vi "Change AO Gain On Fly.vi"() -> ()   [LabVIEW 2015]
doc: "I. Description:\nThis example demonstrates how to output a continuous periodic waveform using an internal sample clock.\n\nII. Instructions for Running:\n1. Select the Physical Channel to correspond to where your signal is output on the DAQ device.\n2. Enter the Minimum and Maximum Voltage Ranges\n3. Specify the Desired Frequency of the output Waveform\n4. Enter the Waveform Information. See the documentation of the Waveform Buffer Generation SubVI for information on each parameter.\n\nIII. Block Diagram Steps:\n1. Create an Analog Output Voltage channel.\n2. Call the DAQmx Timing (Use Waveform) VI which sets the sample clock rate based on the input waveform parameters, and set the sample mode to Continuous.\n3. Write the waveform to the output buffer.\n4. Call the Start VI.\n5. Loop continuously until the user presses the Stop button. Check for errors every 100 ms using the Is Task Done? VI\n6. Clear the Task\n7. Use the popup dialog box to display an error or warning if any.\n\nIV. I/O Connections Overview:\nMake sure your signal output terminal matches the Physical Channel I/O Control. For further connection information, refer to your hardware reference manual."
uses:
  <vilib>/DAQmx/create/channels.llb/DAQmx Create Channel (AO-Voltage-Basic).vi
  <vilib>/Utility/error.llb/DialogType.ctl
  <vilib>/DAQmx/configure/timing.llb/DAQmx Timing (Sample Clock).vi
  <vilib>/DAQmx/write.llb/DAQmx Write (Analog 2D I32 NChan NSamp).vi
panel:
  in  "AO Channel":u16(ring)=1536 items=["AO 0"=1536, "AO 1"=1540]
  in  "Gain Setting":u16(ring) items=["0 dB Gain"=0, "20 dB Gain"=2, "40 dB Gain"=4]
  out "Resulting Frequency":dbl format="%.2f"
  in  "Cycles per Buffer":i32=5
  in  "Waveform Type":T1(ring)
  in  "Desired Frequency":dbl=1000.0 format="%.2f"
  in  "Samples per Buffer":dbl=250.0
  in  "Amplitude":dbl=1750000000.0 format="%0.2p"
  out "Waveform Graph":i32[](graph) caption="Output Waveform"
  in  "Physical Channels":tag="PXI1Slot2/ao0:1"
  in  "Minimum Value":dbl=-10.0 format="%0.2f"
  in  "Maximum Value":dbl=10.0 format="%0.2f"
  in  "stop":bool
  # "For instructions, select Help>>Show Context Help"
  # "Channel Parameters"
  # "Timing Parameters"
  # "Waveform Information"
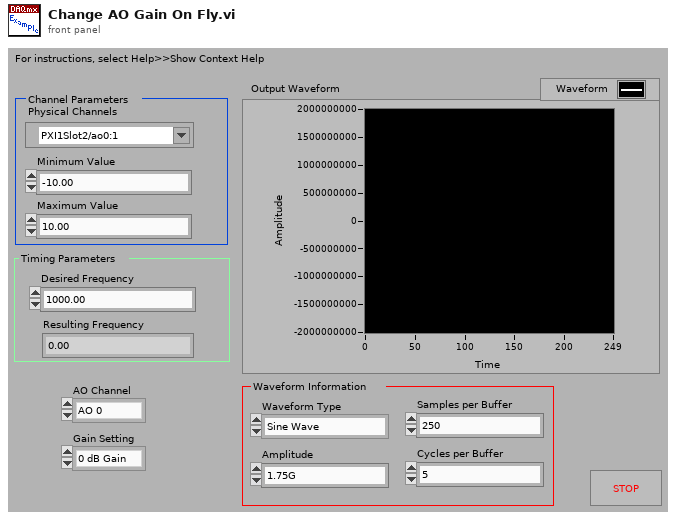
[diagram p1: front panel]
types:
  T1 = enum16{"Sine Wave", "Triangle Wave", "Square Wave", "Sawtooth Wave"}
  T2 = typedef "DialogType.ctl" = u16
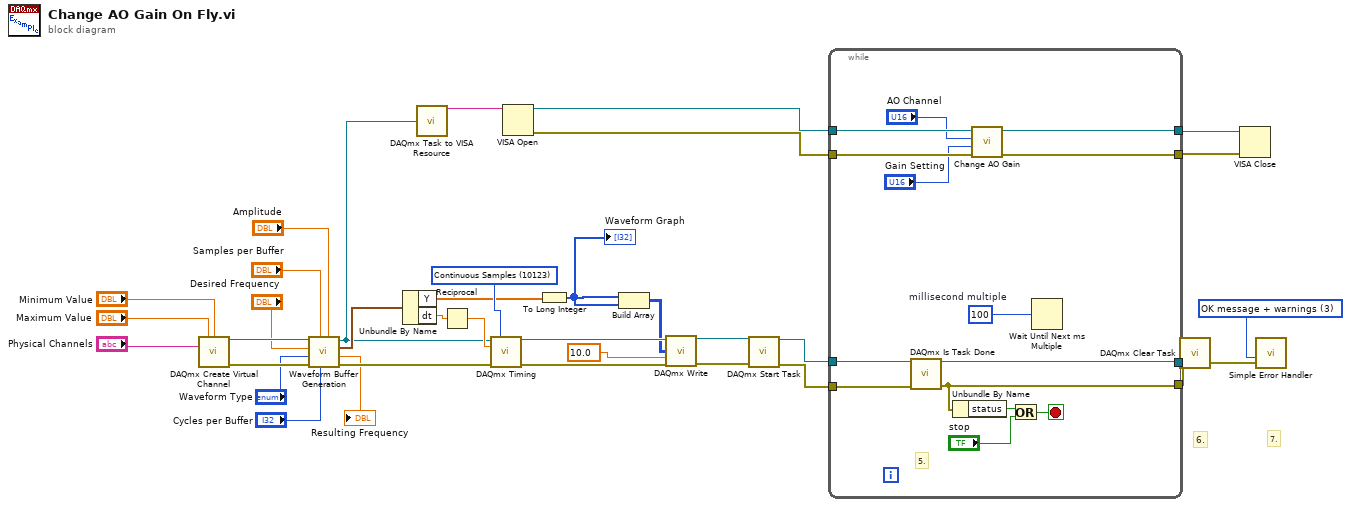
[diagram p0: block diagram]
diagram:
  w6 = 10123 items=["Finite Samples"=10178, "Continuous Samples"=10123, "Hardware Timed Single Point"=12522] ("sample mode")
  w25 = T2 3 items=["no dialog", "OK message", "continue or stop message", "OK message + warnings", "continue/stop + warnings"] ("type of dialog (OK msg:1)")
  # "7."
  # "6."
  n1 = call-poly <vilib>:"DAQmx Create Virtual Channel.vi"("maximum value"="Maximum Value", "minimum value"="Minimum Value", "physical channels"="Physical Channels") -> ("task out"=w21:refnum<k21>, "error out"=w20:errorcluster)  [unwired: 11 in]
  n2 = call "Waveform Buffer Generation.vi"("Amplitude"="Amplitude", "Cycles per Buffer"="Cycles per Buffer", "Samples per Buffer"="Samples per Buffer", "error in (no error)"=w20, "Waveform Type"="Waveform Type", "Desired Frequency"="Desired Frequency", "task/channels in"=w21) -> ("error out"=w22:errorcluster, "Resulting Frequency"=→"Resulting Frequency":dbl, "Waveform"=w9:waveform(dbl), "task out"=w1:refnum<k21>)  [unwired: 1 out]
  n3 = Unbundle By Name(w9) -> ("Y"=w2:dbl[], "dt"=w8:dbl)
  n4 = call "DAQmx Task to VISA Resource.vi"("task out"=w1) -> ("VISAName"=w14:string)
  n5 = Reciprocal(x=w8) -> (1/x=w7:dbl)
  n6 = call-poly <vilib>:"DAQmx Timing.vi"("task/channels in"=w1, "sample mode"=w6, "rate"=w7, "error in"=w22) -> ("task out"=w28:refnum<k21>, "error out"=w27:errorcluster)  [unwired: 10 in]
  n7 = VISA Open(VISA resource name=w14) -> (VISA resource name=w13:refnum<visa-resource-name>, error out=w12:errorcluster)  [unwired: 4 in]
  n8 = To Long Integer(number=w2) -> (32bit integer=w3:i32[])
  "Waveform Graph" <- w3
  n9 = Build Array(w3, w3) -> (w5:i32[][])
  n10 = call-poly <vilib>:"DAQmx Write.vi"("task/channels in"=w28, "data"=w5, "timeout"=10.0 ("Wirite Timeout"), "error in"=w27) -> ("task out"=w33:refnum<k21>, "error out"=w32:errorcluster)  [unwired: 9 in, 1 out]
  n11 = call <vilib>:"DAQmx Start Task.vi"("task/channels in"=w33, "error in"=w32) -> ("task out"=w26:refnum<k21>, "error out"=w30:errorcluster)  [unwired: 12 in]
  n12 = while {
    tunnel: w26 -> [w50]
    tunnel: [w49] -> w24
    tunnel: w30 -> [w48]
    tunnel: [w47] -> w23
    tunnel: w13 -> [w42]
    tunnel: w12 -> [w41]
    tunnel: [w40] -> w11
    tunnel: [w39] -> w10
    stop <- w45 stop-if-true
    w46 = u32 100  # millisecond multiple
    # "5."
    n13 = call <vilib>:"DAQmx Is Task Done.vi"("task/channels in"=w50, "error in"=w48) -> ("task out"=w49:refnum<k21>, "error out"=w47:errorcluster)  [unwired: 11 in, 1 out]
    n14 = Unbundle By Name(w47) -> ("status"=w44:bool)
    n15 = call "Change AO Gain.vi"("error in"=w41, "Gain Setting"="Gain Setting", "AO Channel"="AO Channel", "VISA resource name 2"=w42) -> ("error out"=w39:errorcluster, "VISA resource name"=w40:refnum<visa-resource-name>)  [unwired: 4 in]
    n16 = Or(x=w44, y="stop") -> (x .or. y?=w45:bool)
    n17 = Wait Until Next ms Multiple(millisecond multiple=w46) -> ()  [unwired: 1 out]
  }
  n18 = call <vilib>:"DAQmx Clear Task.vi"("task in"=w24, "error in"=w23) -> ("error out"=w36:errorcluster)  [unwired: 13 in]
  n19 = VISA Close(VISA resource name=w11, error in (no error)=w10) -> ()  [unwired: 1 out]
  n20 = call <vilib>:"Simple Error Handler.vi"("type of dialog (OK msg:1)"=w25, "error in (no error)"=w36) -> ()  [unwired: 3 in, 5 out]
